vi "Autonomous Independent.vi"   [LabVIEW 2013]
doc: "This VI is called when autonomous begins, and will automatically be terminated when autonomous ends. You can carry out timed or sensor driven robot movement independently without needing to return to the caller."
uses:
  Robot Global Data.vi
panel:
  # "Be sure to right-click and choose Data Operations>>Make Current Value default if you want to save the array values with the VI"
types:
  T1 = typedef "WPI_AnalogChannelDevRef.ctl" = cluster{"DevStatus":errorcluster, "Analog Module":T2, "Analog Channel":T3}
  T2 = typedef "FPGA_TypedefAnalogModule.ctl" = enum16{"Analog Module 1", "Analog Module 2"}
  T3 = typedef "FPGA_AIChannel.ctl" = enum8{"AI 1", "AI 2", "AI 3", "AI 4", "AI 5", "AI 6", "AI 7", "AI 8", "Invalid"}
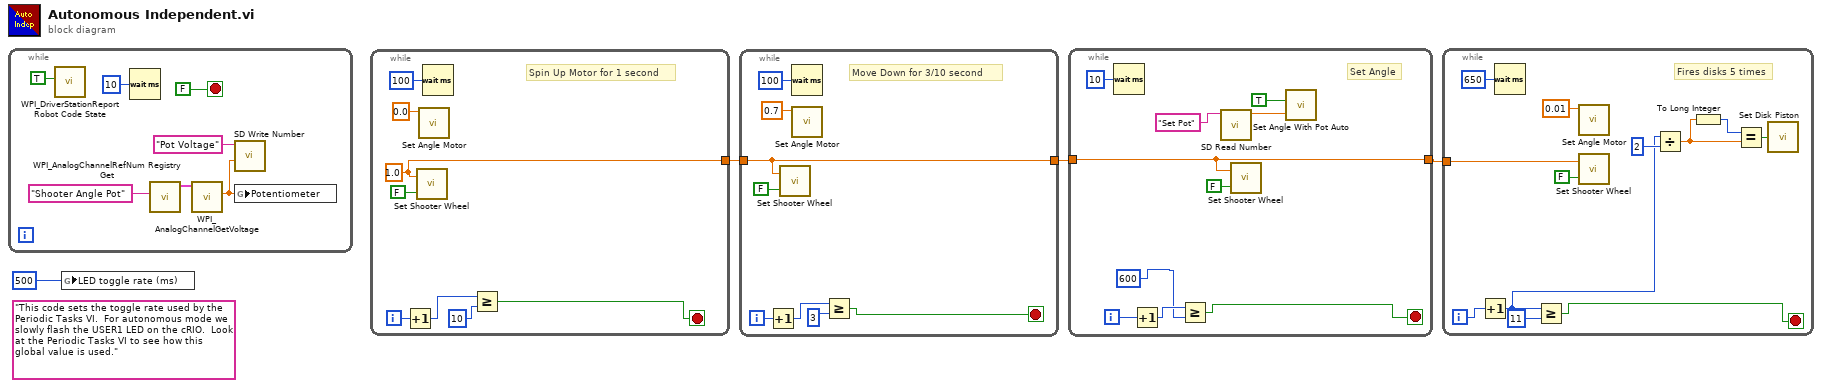
[diagram p0: block diagram]
diagram:
  (unwired) "This code sets the toggle rate used by the Periodic Tasks VI.  For autonomous mode we slowly flash the USER1 LED on the cRIO.  Look at the Periodic Tasks VI to see how this global value is used."
  n1 = while {
    stop <- FALSE stop-if-true
    n2 = call <vilib>:"WPI_DriverStationReport Robot Code State.vi"("Autonomous"=TRUE) -> ()  [unwired: 10 in, 1 out]
    n3 = Wait (ms)(milliseconds to wait=u32 10) -> ()  [unwired: 1 out]
    n4 = call <vilib>:"WPI_AnalogChannelRefNum Registry Get.vi"("refnum name"="Shooter Angle Pot") -> ("AIDeviceRef"=w7:T1)  [unwired: 9 in, 1 out]
    n5 = call <vilib>:"WPI_AnalogChannelGetVoltage.vi"("AIDeviceRef"=w7) -> ("Voltage"=w5:dbl)  [unwired: 8 in, 2 out]
    n6 = call <vilib>:"SD Write Number.vi"("Numeric"=w5, "Name"="Pot Voltage") -> ()  [unwired: 8 in, 2 out]
    n7 = global write "Robot Global Data.vi" "Potentiometer"(w5) -> ()
  }
  n8 = global write "Robot Global Data.vi" "LED toggle rate (ms)"(u32 500 ("LED ms toggle rate")) -> ()
  n9 = while {
    tunnel: [w12] -> w1
    i -> [w18]
    stop <- w15 stop-if-true
    w12 = 1.0 ("Motor Speed")
    # "Spin Up Motor for 1 second"
    n10 = Increment(x=w18) -> (x+1=w17:i32)
    n11 = call "Set Shooter Wheel.vi"("Reverse"=FALSE, "Motor Speed"=w12) -> ()  [unwired: 2 in]
    n12 = call "Set Angle Motor.vi"("Motor Speed"=0.0) -> ()  [unwired: 11 in]
    n13 = Wait (ms)(milliseconds to wait=u32 100) -> ()  [unwired: 1 out]
    n14 = Greater Or Equal?(x=w17, y=10) -> (x >= y?=w15:bool)
  }
  n15 = while {
    tunnel: [w20] -> w3
    tunnel: w1 -> [w20]
    i -> [w26]
    stop <- w23 stop-if-true
    # "Move Down for 3/10 second"
    n16 = Increment(x=w26) -> (x+1=w25:i32)
    n17 = call "Set Shooter Wheel.vi"("Reverse"=FALSE, "Motor Speed"=w20) -> ()  [unwired: 2 in]
    n18 = Wait (ms)(milliseconds to wait=u32 100) -> ()  [unwired: 1 out]
    n19 = call "Set Angle Motor.vi"("Motor Speed"=0.7) -> ()  [unwired: 11 in]
    n20 = Greater Or Equal?(x=w25, y=3) -> (x >= y?=w23:bool)
  }
  n21 = while {
    tunnel: [w32] -> w2
    tunnel: w3 -> [w32]
    i -> [w36]
    stop <- w34 stop-if-true
    # "Set Angle"
    n22 = Wait (ms)(milliseconds to wait=u32 10) -> ()  [unwired: 1 out]
    n23 = Increment(x=w36) -> (x+1=w35:i32)
    n24 = Greater Or Equal?(x=w35, y=600) -> (x >= y?=w34:bool)
    n25 = call <vilib>:"SD Read Number.vi"("Name"="Set Pot" ("refnum name")) -> ("Numeric"=w28:dbl)  [unwired: 8 in, 2 out]
    n26 = call "Set Shooter Wheel.vi"("Reverse"=FALSE, "Motor Speed"=w32) -> ()  [unwired: 2 in]
    n27 = call "Set Angle With Pot Auto.vi"("Set Angle"=w28, "Enable"=TRUE) -> ()  [unwired: 1 in]
  }
  n28 = while {
    tunnel: w2 -> [w39]
    i -> [w48]
    stop <- w46 stop-if-true
    # "Fires disks 5 times"
    n29 = Increment(x=w48) -> (x+1=w41:i32)
    n30 = Wait (ms)(milliseconds to wait=u32 650) -> ()  [unwired: 1 out]
    n31 = Greater Or Equal?(x=w41, y=11) -> (x >= y?=w46:bool)
    n32 = call "Set Angle Motor.vi"("Motor Speed"=0.01) -> ()  [unwired: 11 in]
    n33 = call "Set Shooter Wheel.vi"("Reverse"=FALSE, "Motor Speed"=w39) -> ()  [unwired: 2 in]
    n34 = Divide(x=w41, y=2) -> (x/y=w44:dbl)
    n35 = To Long Integer(number=w44) -> (32bit integer=w43:i32)
    n36 = Equal?(x=w43, y=w44) -> (x = y?=w40:bool)
    n37 = call "Set Disk Piston.vi"("Boolean"=w40) -> ()
  }
